vi "Connect Error Wire If not Connected.vi"(8 "error in (no error)":errorcluster, 10 "case":string, 11 "CSM-Helper in":refnum<class "CSM-Helper.lvclass">) -> (0 "error out":errorcluster, 3 "CSM-Helper out":refnum<class "CSM-Helper.lvclass">)   [LabVIEW 2017, in "CSM-Helper.lvclass"]
doc: "### Connect Error Wire If not Connected.vi\n\n-- <b>Controls</b> --\n- <b>case</b>:\n- <b>CSM-Helper in</b>: CSMHelper input\n\n-- <b>Indicators</b> --\n- <b>CSM-Helper out</b>: CSMHelper output"
uses:
  CSM-Helper.lvclass
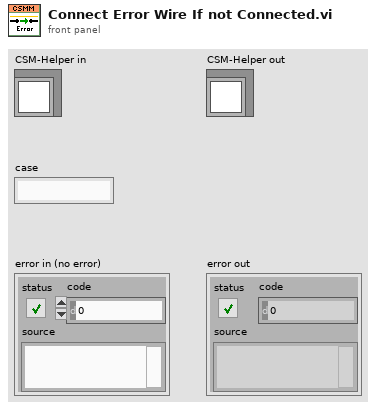
[diagram p1: front panel]
types:
  T1 = cluster{"Registration":refnum<vi>, "InternalData":refnum<vi>, "CSM Name":refnum<vi>, "Last Resp":refnum<vi>, "Remaining State":refnum<vi>, "Arguments":refnum<vi>, "Response Source":refnum<vi>, "Source CSM":refnum<vi>, "Selector":refnum<vi>, "Error":refnum<vi>}
  T2 = cluster{"Registration":refnum<vi>, "InternalData":refnum<vi>, "Resp":refnum<vi>, "Remaining State":refnum<vi>, "Error":refnum<vi>}
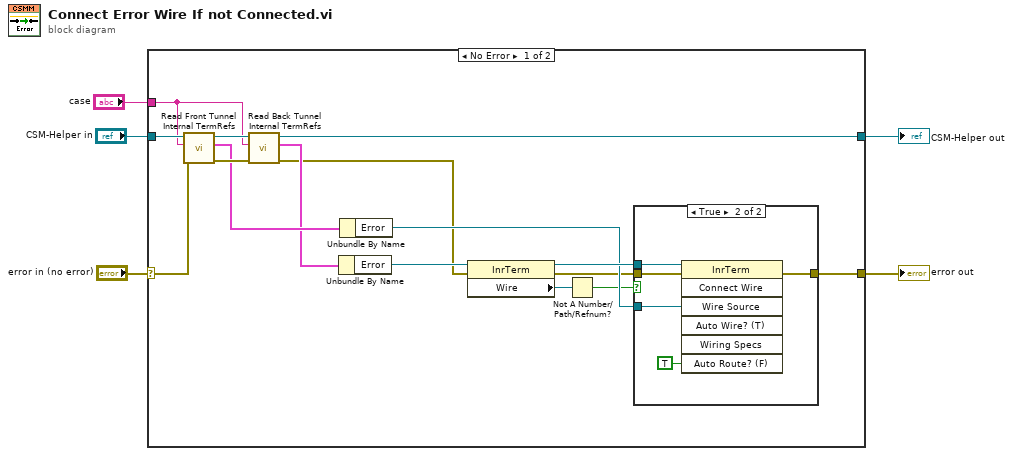
[diagram p0: block diagram]
diagram:
  n1 = case shown="No Error" "error in (no error)" {
    selector: "error in (no error)" -> [w8 w29]
    tunnel: "CSM-Helper in" -> [w10 w28]
    tunnel: [w9 w28] -> w4
    tunnel: [w7 w29] -> w2
    tunnel: "case" -> [w6 _]
    frame No Error {
      n2 = call "Read Front Tunnel Internal TermRefs.vi"("error in (no error)"=w8, "case"=w6, "CSM-Helper in"=w10) -> ("error out"=w20:errorcluster, "Front Tunnels"=w19:T1, "CSM-Helper out"=w21:refnum<class "CSM-Helper.lvclass">)  [unwired: 6 in]
      n3 = call "Read Back Tunnel Internal TermRefs.vi"("error in (no error)"=w20, "element"=w6, "CSM-Helper in"=w21) -> ("error out"=w11:errorcluster, "Back Tunnels"=w17:T2, "CSM-Helper out"=w9:refnum<class "CSM-Helper.lvclass">)  [unwired: 6 in]
      n4 = Unbundle By Name(w17) -> ("Error"=w18:refnum<vi>)
      n5 = Unbundle By Name(w19) -> ("Error"=w14:refnum<vi>)
      n6 = property class="InrTerm"(reference=w18, error in=w11) -> (reference out=w15:refnum<vi>, error out=w12:errorcluster, "Wire"=w16:refnum<vi>)
      n7 = Not A Number/Path/Refnum?(number/path/refnum=w16) -> (NaN/Path/Refnum?=w13:bool)
      n8 = case shown="True" w13 {
        tunnel: w15 -> [_ w27]
        tunnel: w14 -> [_ w26]
        tunnel: w12 -> [w22 w24]
        tunnel: [w22 w23] -> w7
        frame False {
        }
        frame True {
          n9 = invoke class="InrTerm" method="Connect Wire"(reference=w27, error in=w24, "Wire Source"=w26, "Auto Route? (F)"=TRUE) -> (error out=w23:errorcluster)  [unwired: 3 in, 6 out]
        }
      }
    }
    frame Error {
    }
  }
  "CSM-Helper out" <- w4
  "error out" <- w2
